vi "Subscribe to Request-Reply.vi"(8 "error in (no error)":errorcluster, 11 "Example Request in":refnum<k1>) -> (0 "error out":errorcluster, 2 "Request-Reply Registration":refnum<event-registration>, 3 "Example Request out":refnum<k1>)   [LabVIEW 2018, in "Actor.lvclass"]
uses:
  Actor.lvclass
  Example-Request.ctl
  Example-Reply.ctl
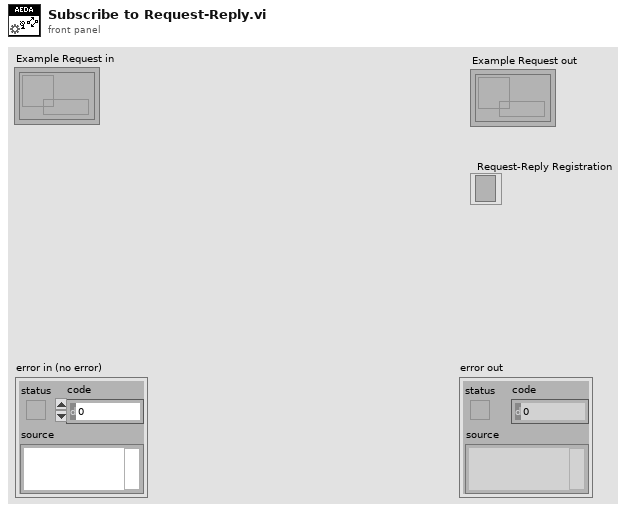
[diagram p1: front panel]
types:
  T1 = typedef "Actor.lvclass/Example-Request.ctl" = cluster{"Number":bool, "String":string}
  T2 = cluster{"Example-Request":refnum<user-event>, "event data":cluster{"Number":T1, "Reply":refnum<user-event>}}
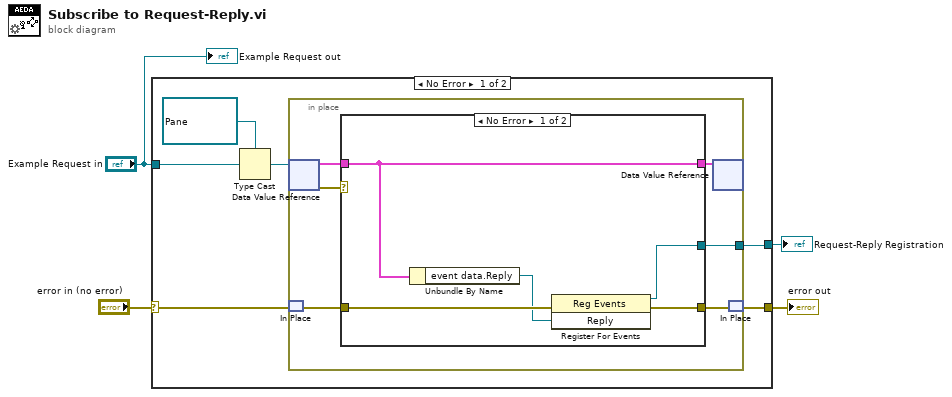
[diagram p0: block diagram]
diagram:
  n1 = case shown="No Error" "error in (no error)" {
    selector: "error in (no error)" -> [w10 w24]
    tunnel: [w9 w24] -> w3
    tunnel: "Example Request in" -> [w8 _]
    tunnel: [w5 _] -> w1
    frame No Error {
      n2 = Type Cast(type=refnum<data-value> refnum ("data value reference"), x=w8) -> (*(type *) &x=w7:refnum<data-value>)
      n3 = in-place {
        in-place-border: [w11] -> w5
        n4 = in-place-dvr #1(w7) -> (w15:T2, w16:errorcluster)
        n5 = in-place-match #2(w10) -> (w13:errorcluster)
        n6 = case shown="No Error" w16 {
          selector: w16 -> [_ w23]
          tunnel: w15 -> [w21 w22]
          tunnel: [w21 w22] -> w14
          tunnel: w13 -> [w20 _]
          tunnel: [w18 w23] -> w12
          tunnel: [w17 _] -> w11
          frame No Error {
            n7 = Unbundle By Name(w21) -> ("event data.Reply"=w19:refnum<user-event>)
            n8 = register-events(error in=w20, w19) -> (reference out=w17:refnum<event-registration>, error out=w18:errorcluster)  [unwired: 1 in]
          }
          frame Error {
          }
        }
        n9 = in-place-dvr #1(w14) -> ()  [unwired: 2 out]
        n10 = in-place-match #2(w12) -> (w9:errorcluster)
      }
    }
    frame Error {
    }
  }
  "error out" <- w3
  "Request-Reply Registration" <- w1
  "Example Request out" <- "Example Request in"
